vi "Handle getAll.vi"(8 "error in (no error)":errorcluster, 11 "Instrument.Oxford1820 in":refnum<class "Instrument.Oxford1820.lvclass">) -> (0 "error out":errorcluster, 2 "getAll":variant, 3 "Instrument.Oxford1820 out":refnum<class "Instrument.Oxford1820.lvclass">)   [LabVIEW 2019, in "Instrument.Oxford1820.lvclass"]
uses:
  Instrument.Oxford1820.lvclass
  Instrument.Oxford1820.lvclass/Instrument.Oxford1820.ctl
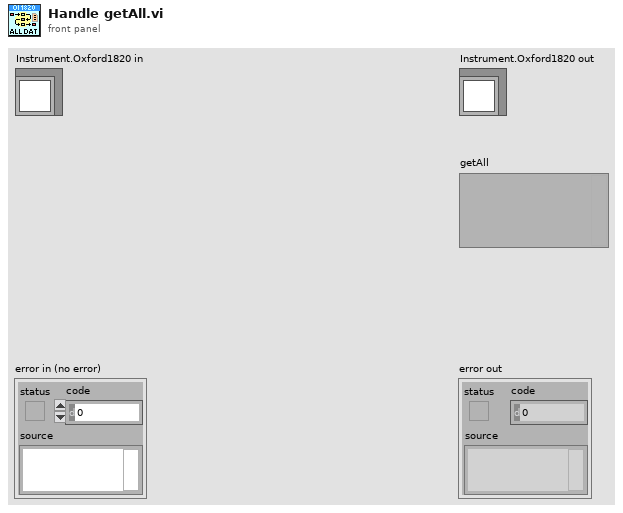
[diagram p1: front panel]
types:
  T1 = typedef "Instrument.Oxford1820.lvclass/getAll.ctl" = cluster{"1820_IPS_Magnet_Field":dbl, "1820_IPS_PS_Field":dbl, "1820_IPS_Target_Field":dbl, "1820_IPS_Target_Field_Rate":dbl, "1820_IPS_Voltage":dbl, "1820_IPS_Current":dbl, "1820_IPS_Level_N2":dbl, "1820_IPS_Level_He":dbl, "1820_IPS_Magnet_Temperature":dbl, "1820_IPS_Magnet_Temperature_R":dbl, "1820_IPS_M1_Current":dbl, "1820_IPS_M1_Voltage":dbl, "1820_IPS_M2_Current":dbl, "1820_IPS_M2_Voltage":dbl, "1820_IPS_M3_Current":dbl, "1820_IPS_M3_Voltage":dbl, "1820_IPS_Status":string, "1820_IPS_Switch":string, "1820_ITC_Lambda_Temperature":dbl, "1820_ITC_Lambda_Temperature_R":dbl, "1820_ITC_Pressure":dbl, "1820_ITC_Needle_Valve":dbl}
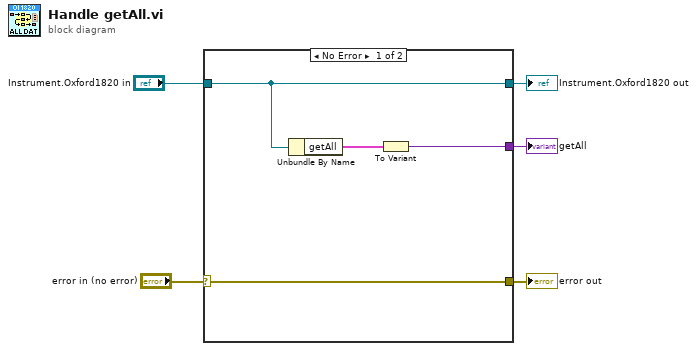
[diagram p0: block diagram]
diagram:
  n1 = case shown="No Error" "error in (no error)" {
    selector: "error in (no error)" -> [w7 w10]
    tunnel: "Instrument.Oxford1820 in" -> [w6 w11]
    tunnel: [w6 w11] -> w4
    tunnel: [w7 w10] -> w2
    tunnel: [w8 _] -> w1
    frame No Error {
      n2 = Unbundle By Name(w6) -> ("getAll"=w9:T1)
      n3 = To Variant(anything=w9) -> (Variant=w8:variant)
    }
    frame Error {
    }
  }
  "error out" <- w2
  "Instrument.Oxford1820 out" <- w4
  "getAll" <- w1
